vi "Initialize.vi"(7 "Channel Name":string="Setpoint.ch%d.SP", 8 "error in":errorcluster, 9 "Number of Channels":u32=1, 10 "Instance Name":string="PluginName", 11 "Temperature Gradient in":refnum<class "Temperature Gradient.lvclass">) -> (0 "error out":errorcluster, 3 "Temperature Gradient out":refnum<class "Temperature Gradient.lvclass">)   [LabVIEW 2023, in "Temperature Gradient.lvclass"]
uses:
  Temperature Gradient.lvclass
  Temperature Gradient.lvclass/Temperature Gradient.ctl
  Parents/Gradient/Gradient.lvclass
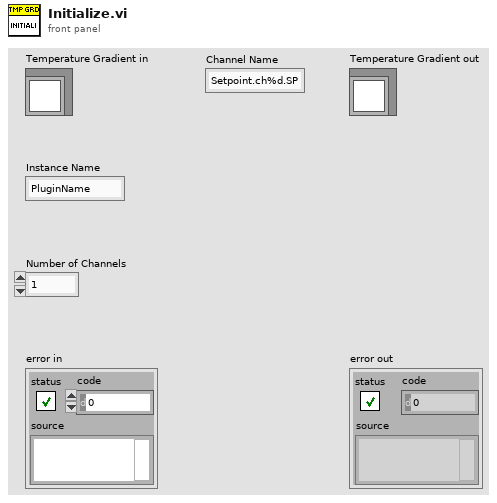
[diagram p1: front panel]
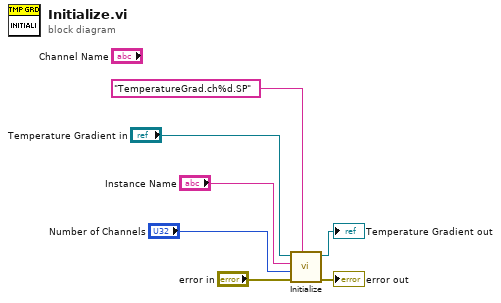
[diagram p0: block diagram]
diagram:
  n1 = call-parent "Initialize.vi"("Channel Name"="TemperatureGrad.ch%d.SP" ("ChannelName"), "error in"="error in", "Number of Channels"="Number of Channels", "Instance Name"="Instance Name", "Gradient in"="Temperature Gradient in") -> ("error out"=→"error out":errorcluster, "Gradient out"=→"Temperature Gradient out":refnum<class "Temperature Gradient.lvclass">)  [unwired: 5 in]
